vi "S-Curve.vi"(9 "dt (s)":dbl=1.0, 10 "goal":dbl, 11 "Limits":T1) -> (0 "X":dbl[](array[numeric]), 1 "T":dbl[](array[numeric]), 2 "A":dbl[](array[numeric]), 3 "V":dbl[](array[numeric]))   [LabVIEW 2019]
panel:
  out "output variable":dbl
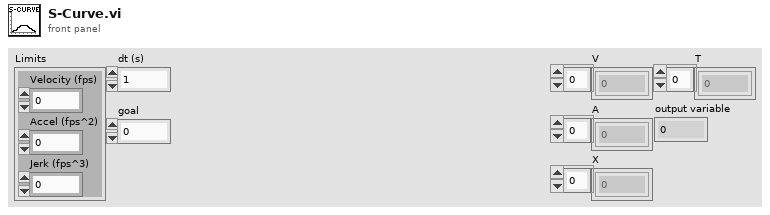
[diagram p1: front panel]
types:
  T1 = cluster{"Velocity (fps)":dbl, "Accel (fps^2)":dbl, "Jerk (fps^3)":dbl}
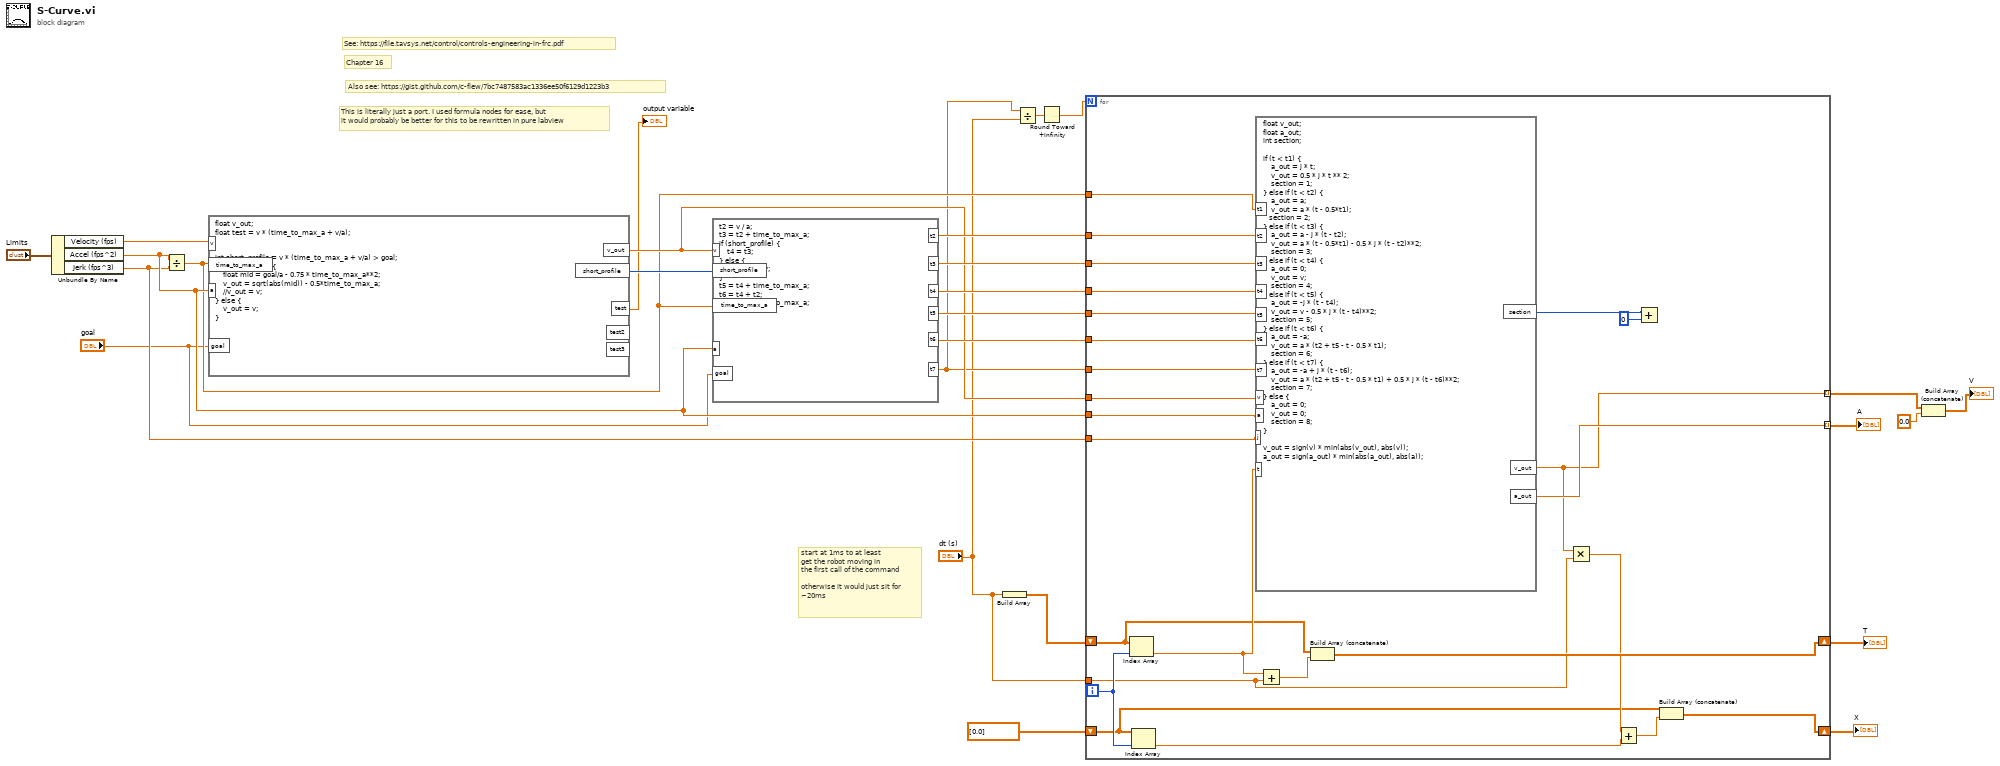
[diagram p0: block diagram]
diagram:
  # "This is literally just a port. I used formula nodes for ease, but\nit would probably be better for this to be rewritten in pure labview"
  # "Also see: https://gist.github.com/c-flew/7bc7487583ac1336ee50f6129d1223b3"
  # "Chapter 16"
  # "See: https://file.tavsys.net/control/controls-engineering-in-frc.pdf"
  # "start at 1ms to at least\nget the robot moving in\nthe first call of the command\n\notherwise it would just sit for \n~20ms"
  n1 = Unbundle By Name("Limits") -> ("Velocity (fps)"=w25:dbl, "Accel (fps^2)"=w17:dbl, "Jerk (fps^3)"=w16:dbl)
  n2 = Divide(x=w17, y=w16) -> (x/y=w15:dbl)
  n3 = formula code="float v_out;\nfloat test = v * (time_to_max_a + v/a);\n\n\nint short_profile = v * (time_to_max_a + v/a) > goal;\nif (short_profile) {\n    float mid = goal/a - 0.75 * time_to_max_a**2;\n    v_out = sqrt(abs(mid)) - 0.5*time_to_max_a;\n    //v_out = v;\n} else {\n    v_out = v;\n}"("goal"="goal", "time_to_max_a"=w15, "v"=w25, "a"=w17) -> ("v_out"=w18:dbl, "short_profile"=w24:i32, "test"=→"output variable":dbl)  [unwired: 2 out]
  n4 = formula code="t2 = v / a;\nt3 = t2 + time_to_max_a;\nif (short_profile) {\n    t4 = t3;\n} else {\n    t4 = goal / v;\n}\nt5 = t4 + time_to_max_a;\nt6 = t4 + t2;\nt7 = t6 + time_to_max_a;"("short_profile"=w24, "v"=w18, "a"=w17, "time_to_max_a"=w15, "goal"="goal") -> ("t2"=w23:dbl, "t3"=w22:dbl, "t4"=w21:dbl, "t5"=w20:dbl, "t6"=w19:dbl, "t7"=w4:dbl)
  n5 = Build Array("dt (s)") -> (w5:dbl[])
  n6 = Divide(x=w4, y="dt (s)") -> (x/y=w2:dbl)
  n7 = Round Toward +Infinity(x=w2) -> (ceil(x): smallest int >= x=w1:dbl)
  n8 = for {
    N: w1 -> [_]
    tunnel: w23 -> [w51]
    tunnel: w22 -> [w50]
    tunnel: w21 -> [w49]
    tunnel: w20 -> [w48]
    tunnel: w19 -> [w47]
    tunnel: w4 -> [w46]
    tunnel: w18 -> [w45]
    tunnel: w17 -> [w44]
    tunnel: w16 -> [w43]
    shift-right: [w35] -> w13
    shift-left: w5 -> [w37]
    tunnel: w15 -> [w42]
    tunnel: [w33] -> w8 mode=indexing
    tunnel: [w41] -> w14 mode=indexing
    shift-right: [w28] -> w10
    shift-left: dbl[] [0.0] ("appended array") -> [w30]
    tunnel: "dt (s)" -> [w27]
    i -> [w34]
    n9 = Index Array(array=w37, index=w34) -> (element=w38:dbl)
    n10 = Index Array(array=w30, index=w34) -> (element=w31:dbl)
    n11 = formula code="float v_out;\nfloat a_out;\nint section;\n\nif (t < t1) {\n    a_out = j * t;\n    v_out = 0.5 * j * t ** 2;\n    section = 1;\n} else if (t < t2) {\n    a_out = a;\n    v_out = a * (t - 0.5*t1);\n   section = 2;\n} else if (t < t3) {\n    a_out = a - j * (t - t2);\n    v_out = a * (t - 0.5*t1) - 0.5 * j * (t - t2)**2;\n    section = 3;\n} else if (t < t4) {\n    a_out = 0;\n    v_out = v;\n    section = 4;\n} else if (t < t5) {\n    a_out = -j * (t - t4);\n    v_out = v - 0.5 * j * (t - t4)**2;\n    section = 5;\n} else if (t < t6) {\n    a_out = -a;\n    v_out = a * (t2 + t5 - t - 0.5 * t1);\n    section = 6;\n} else if (t < t7) {\n    a_out = -a + j * (t - t6);\n    v_out = a * (t2 + t5 - t - 0.5 * t1) + 0.5 * j * (t - t6)**2;\n    section = 7;\n} else {\n    a_out = 0;\n    v_out = 0;\n    section = 8;\n}\n\nv_out = sign(v) * min(abs(v_out), abs(v));\na_out = sign(a_out) * min(abs(a_out), abs(a));"("t2"=w51, "t3"=w50, "t4"=w49, "t5"=w48, "t6"=w47, "t7"=w46, "v"=w45, "a"=w44, "j"=w43, "t"=w38, "t1"=w42) -> ("v_out"=w33:dbl, "a_out"=w41:dbl, "section"=w40:i32)
    n12 = Add(x=w38, y=w27) -> (x+y=w36:dbl)
    n13 = Build Array (concatenate)(w37, w36) -> (w35:dbl[])
    n14 = Multiply(x=w33, y=w27) -> (x*y=w32:dbl)
    n15 = Add(x=w32, y=w31) -> (x+y=w29:dbl)
    n16 = Add(x=w40, y=0) -> ()  [unwired: 1 out]
    n17 = Build Array (concatenate)(w30, w29) -> (w28:dbl[])
  }
  "A" <- w14
  "T" <- w13
  "X" <- w10
  n18 = Build Array (concatenate)(w8, 0.0 ("output variable")) -> (→"V":dbl[])
